vi "PTScanner.ProcEvents.vi"(0 "i ref in":refnum<vi>, 5 "error in":errorcluster) -> (14 "i ref out":refnum<vi>, 19 "error out":errorcluster)   [LabVIEW 2014, in "PTScanner.lvlib"]
uses:
  PTScanner.lvlib
  CS_Core/BaseProcess/BaseProcess.event definition.ctl
  CS_Core/CAEObj/CAEObj.event definition.ctl
  CS_Core/BaseProcess/BaseProcess.descriptor string definition.ctl
  CS_Core/BaseProcess/BaseProcess.lvlib
  CS_Core/CAEObj/CAEObj.lvlib
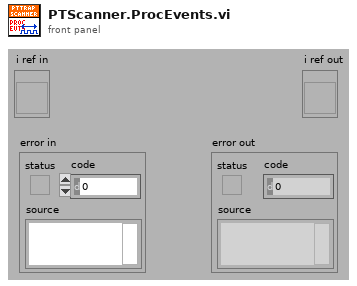
[diagram p1: front panel]
types:
  T1 = typedef "BaseProcess.lvlib/BaseProcess.event definition.ctl" = cluster{"CAEEvtDef":T2, "Data Descriptor":T3}
  T2 = typedef "CAEObj.lvlib/CAEObj.event definition.ctl" = cluster{"URL":string, "enable":bool, "ignoreResID":bool}
  T3 = typedef "BaseProcess.lvlib/BaseProcess.descriptor string definition.ctl" = string
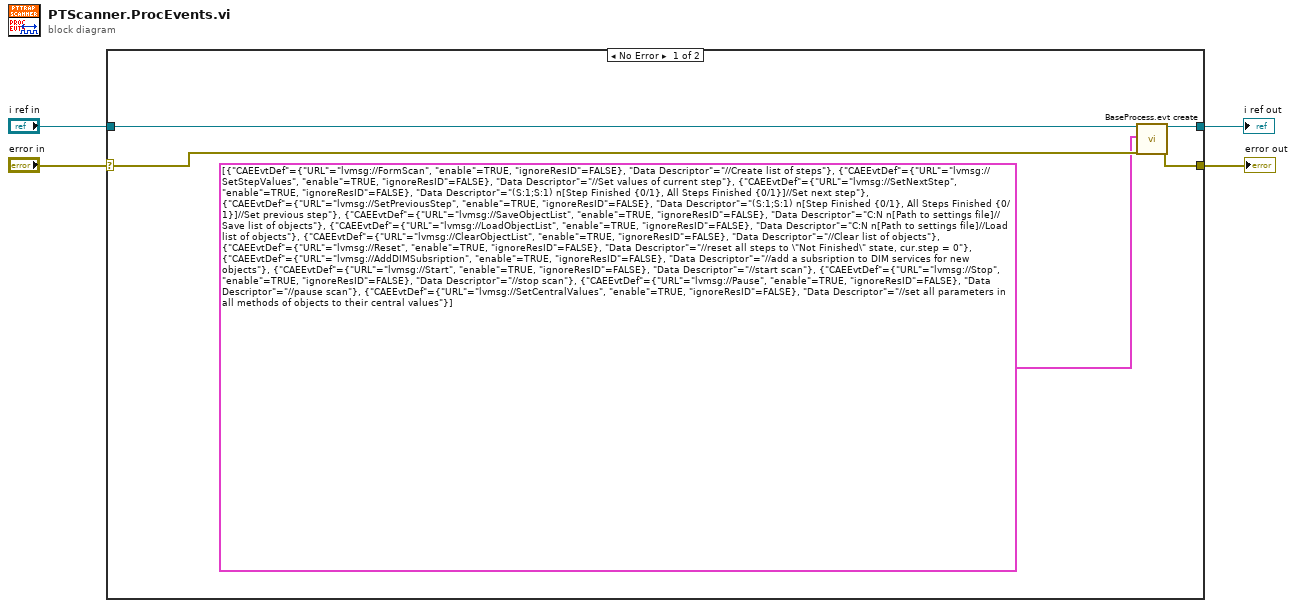
[diagram p0: block diagram]
diagram:
  n1 = case shown="No Error" "error in" {
    selector: "error in" -> [w7 w10]
    tunnel: "i ref in" -> [w6 w11]
    tunnel: [w9 w11] -> w3
    tunnel: [w8 w10] -> w2
    frame No Error {
      n2 = call "BaseProcess.evt create.vi"("i ref in"=w6, "newEvents"=T1[] [{"CAEEvtDef"={"URL"="lvmsg://FormScan", "enable"=TRUE, "ignoreResID"=FALSE}, "Data Descriptor"="//Create list of steps"}, {"CAEEvtDef"={"URL"="lvmsg://SetStepValues", "enable"=TRUE, "ignoreResID"=FALSE}, "Data Descriptor"="//Set values of current step"}, {"CAEEvtDef"={"URL"="lvmsg://SetNextStep", "enable"=TRUE, "ignoreResID"=FALSE}, "Data Descriptor"="(S:1;S:1) n[Step Finished {0/1}, All Steps Finished {0/1}]//Set next step"}, {"CAEEvtDef"={"URL"="lvmsg://SetPreviousStep", "enable"=TRUE, "ignoreResID"=FALSE}, "Data Descriptor"="(S:1;S:1) n[Step Finished {0/1}, All Steps Finished {0/1}]//Set previous step"}, {"CAEEvtDef"={"URL"="lvmsg://SaveObjectList", "enable"=TRUE, "ignoreResID"=FALSE}, "Data Descriptor"="C:N n[Path to settings file]//Save list of objects"}, {"CAEEvtDef"={"URL"="lvmsg://LoadObjectList", "enable"=TRUE, "ignoreResID"=FALSE}, "Data Descriptor"="C:N n[Path to settings file]//Load list of objects"}, {"CAEEvtDef"={"URL"="lvmsg://ClearObjectList", "enable"=TRUE, "ignoreResID"=FALSE}, "Data Descriptor"="//Clear list of objects"}, {"CAEEvtDef"={"URL"="lvmsg://Reset", "enable"=TRUE, "ignoreResID"=FALSE}, "Data Descriptor"="//reset all steps to \"Not Finished\" state, cur.step = 0"}, {"CAEEvtDef"={"URL"="lvmsg://AddDIMSubsription", "enable"=TRUE, "ignoreResID"=FALSE}, "Data Descriptor"="//add a subsription to DIM services for new objects"}, {"CAEEvtDef"={"URL"="lvmsg://Start", "enable"=TRUE, "ignoreResID"=FALSE}, "Data Descriptor"="//start scan"}, {"CAEEvtDef"={"URL"="lvmsg://Stop", "enable"=TRUE, "ignoreResID"=FALSE}, "Data Descriptor"="//stop scan"}, {"CAEEvtDef"={"URL"="lvmsg://Pause", "enable"=TRUE, "ignoreResID"=FALSE}, "Data Descriptor"="//pause scan"}, {"CAEEvtDef"={"URL"="lvmsg://SetCentralValues", "enable"=TRUE, "ignoreResID"=FALSE}, "Data Descriptor"="//set all parameters in all methods of objects to their central values"}] ("new events"), "error in (no error)"=w7) -> ("i ref out"=w9:refnum<vi>, "error out"=w8:errorcluster)  [unwired: 13 in, 2 out]
    }
    frame Error {
    }
  }
  "i ref out" <- w3
  "error out" <- w2
